vi "Actor Core.vi"(8 "error in":errorcluster, 11 "AlbumImageActor in":refnum<class "AlbumImageActor.lvclass">) -> (0 "error out":errorcluster, 3 "Actor out":refnum<class "Actor.lvclass">)   [LabVIEW 2015, in "AlbumImageActor.lvlib" / "AlbumImageActor.lvclass"]
doc: "(<B>Filename</B>: Actor Framework.lvlib:Actor.lvclass:Actor Core.vi)\n\nReceives messages to the actor, reacts to them, and initiates any error handling that may shut the actor down.\n\nDescendant classes may override this VI to append parallel tasks for the actor to complete while it handles messages. Overrides use the Call Parent Method node."
uses:
  AlbumImageActor.lvclass
  <vilib>/ActorFramework/Actor/Actor.lvclass
  AlbumImageActor.lvclass/AlbumImageActor.ctl
  <vilib>/ActorFramework/Actor/Actor.lvclass/Actor.ctl
  <vilib>/ActorFramework/Message Enqueuer/Message Enqueuer.lvclass/Message Enqueuer.ctl
  <vilib>/ActorFramework/Message Enqueuer/Init from Existing Queue.vi
  <vilib>/ActorFramework/Message Enqueuer/Enqueue.vi
  <vilib>/ActorFramework/Message Priority Queue/Priority Enqueue.vi
  <vilib>/ActorFramework/Message Enqueuer/Message Enqueuer.lvclass
  <vilib>/ActorFramework/Stop Msg/Stop Msg.lvclass
panel:
  out "Album Image":picture
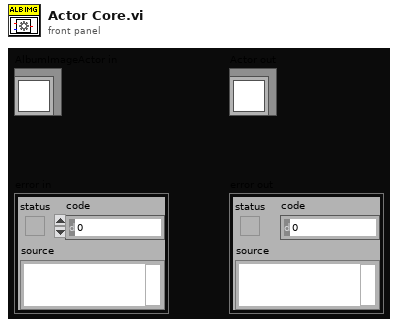
[diagram p1: front panel]
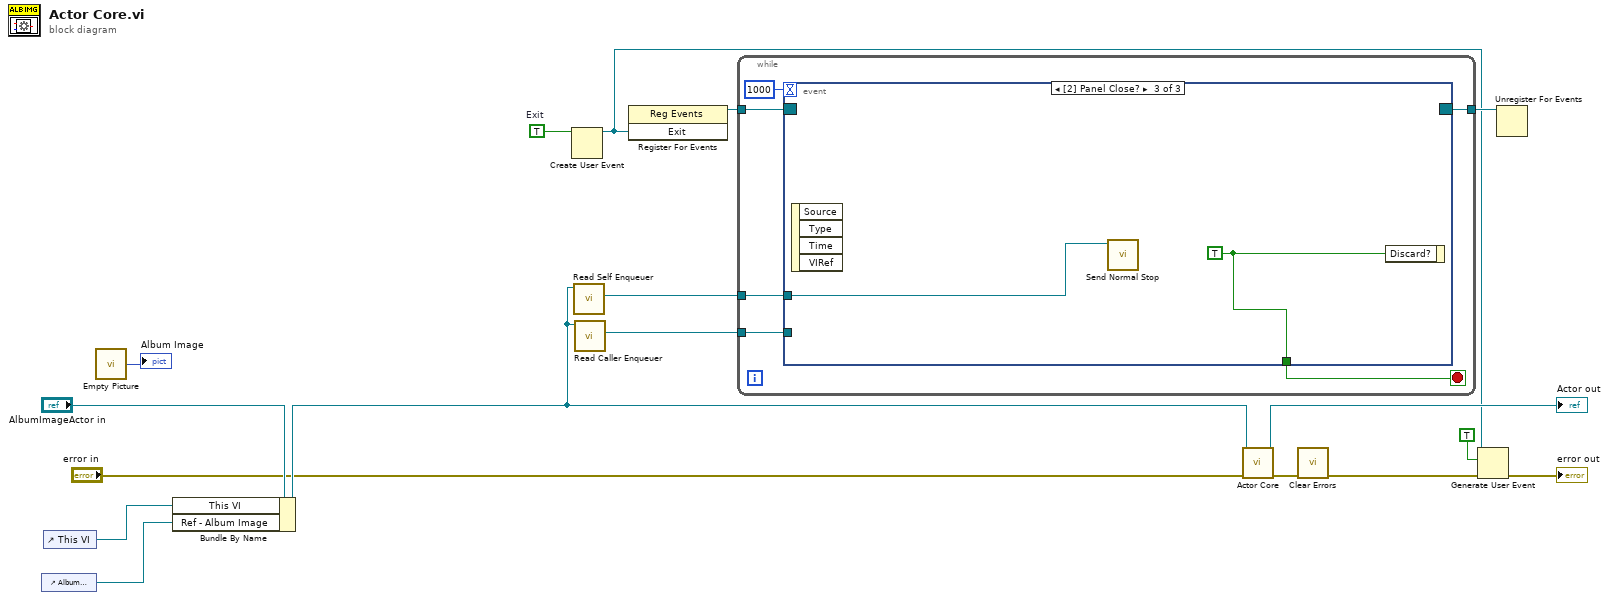
[diagram p0: block diagram]
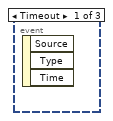
[diagram p2: hidden frame]
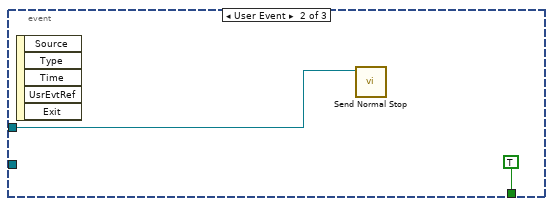
[diagram p3: hidden frame]
diagram:
  w16 = TRUE  # Exit
  n1 = control-ref of="Album Image"() -> (w2:refnum<vi>)
  n2 = control-ref of="This VI"() -> (w4:refnum<vi>)
  n3 = call "Empty Picture"() -> ("empty picture"=→"Album Image":picture)
  n4 = Bundle By Name(cluster="AlbumImageActor in", "This VI"=w4, "Ref - Album Image"=w2) -> (w5:refnum<class "AlbumImageActor.lvclass">)
  n5 = Create User Event(user event datatype=w16) -> (user event=w8:refnum<user-event>)  [unwired: 1 in, 1 out]
  n6 = call <vilib>:"Read Self Enqueuer.vi"("Actor"=w5) -> ("Self Enqueuer"=w9:refnum<class "Message Enqueuer.lvclass">)  [unwired: 10 in]
  n7 = call <vilib>:"Read Caller Enqueuer.vi"("Actor"=w5) -> ("Caller Enqueuer"=w7:refnum<class "Message Enqueuer.lvclass">)  [unwired: 10 in]
  n8 = register-events(w8) -> (reference out=w15:refnum<event-registration>)  [unwired: 2 in, 1 out]
  n9 = while {
    tunnel: w15 -> [w23]
    tunnel: [w21] -> w14
    tunnel: w9 -> [w20]
    tunnel: w7 -> [w18]
    stop <- w22 stop-if-true
    n10 = event shown="[2] Panel Close?" {
      selector: w23 -> [_ _ _]
      dyn-events: [_ _ _] -> w21
      timeout: 1000 -> [_ _ _]
      tunnel: [_ TRUE ("Exit") w27] -> w22
      tunnel: w20 -> [_ w24 w26]
      tunnel: w18 -> [_ _ _]
      event Timeout {
        n11 = event-data() -> ()  [unwired: 1 in, 3 out]
      }
      event User Event {
        n12 = event-data() -> ()  [unwired: 1 in, 5 out]
        n13 = call <vilib>:"Send Normal Stop.vi"("Message Enqueuer"=w24) -> ()  [unwired: 10 in, 1 out]
      }
      event Panel Close? {
        w27 = TRUE ("Discard?")
        n14 = event-data() -> ()  [unwired: 1 in, 4 out]
        n15 = call <vilib>:"Send Normal Stop.vi"("Message Enqueuer"=w26) -> ()  [unwired: 10 in, 1 out]
        n16 = event-data("Discard?"=w27) -> ()  [unwired: 1 in, 1 out]
      }
    }
  }
  n17 = call-parent "Actor Core.vi"("error in"="error in", "Actor in"=w5) -> ("error out"=w13:errorcluster, "Actor out"=→"Actor out":refnum<class "Actor.lvclass">)  [unwired: 8 in]
  n18 = call <vilib>:"Clear Errors.vi"("error in (no error)"=w13) -> ("error out"=w11:errorcluster)  [unwired: 5 in, 1 out]
  n19 = Generate User Event(user event=w8, event data cluster=TRUE ("event data"), error in=w11) -> (error out=→"error out":errorcluster)  [unwired: 1 in, 1 out]
  n20 = Unregister For Events(event registration refnum=w14) -> ()  [unwired: 1 in, 1 out]
